vi "Acquisition Status.vi"(8 "error in (no error)":errorcluster {"code" format="%.0x"}, 11 "instrument handle":refnum<k15>) -> (0 "error out":errorcluster {"code" format="%.0x"}, 1 "acquisition status":i32 format="%.0g", 3 "instrument handle out":refnum<k15>)   [LabVIEW 2009, in "Keysight XSAn.lvlib"]
doc: "This function determines if an acquisition is in progress or complete.\n\nSupported Models: All supported"
uses:
  <instrlib>/Keysight XSAn/Keysight XSAn.lvlib
  AgXSAn.dll
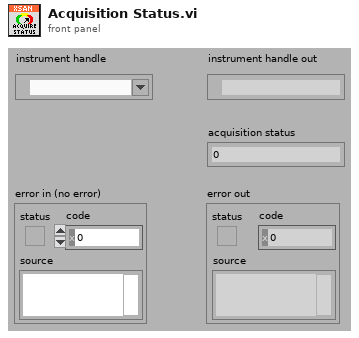
[diagram p1: front panel]
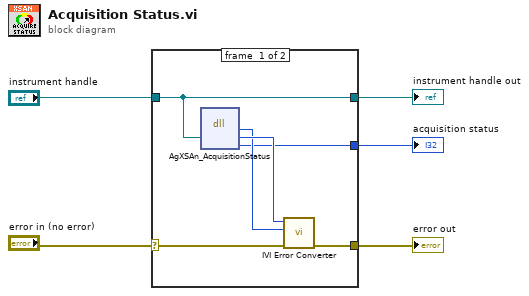
[diagram p0: block diagram]
diagram:
  n1 = case shown="No Error" "error in (no error)" {
    selector: "error in (no error)" -> [w9 w13]
    tunnel: [w10 w13] -> w4
    tunnel: "instrument handle" -> [w6 w12]
    tunnel: [w7 _] -> w2
    tunnel: [w6 w12] -> w1
    frame #0 {
      n2 = dll-call lib="AgXSAn**.dll" fn="AgXSAn_AcquisitionStatus" ("LabVIEW:IviSpecAn_AcquisitionStatus")("instrument handle"=w6) -> ("Status"=w8:i32, "instrument handle"=w11:u32, "acquisition status"=w7:i32)  [unwired: 3 in, 3 out]
      n3 = call <instrlib>:"IVI Error Converter.vi"("error in (no error)"=w9, "IVI error code (0)"=w8, "instrument handle"=w11) -> ("error out"=w10:errorcluster)  [unwired: 7 in, 1 out]
    }
    frame #1 {
    }
  }
  "error out" <- w4
  "instrument handle out" <- w1
  "acquisition status" <- w2
